vi "determinateTheRawSizeOfTable.vi"(0 "tableName":string, 3 "error in":errorcluster) -> (7 "sizeOfTableInNumberRaw":i32, 10 "error out":errorcluster)   [LabVIEW 2014]
uses:
  <vilib>/addons/database/Connection.llb/DB Tools Open Connec (String).vi
  <vilib>/addons/database/Connection.llb/Conn Execute.vi
  <vilib>/addons/database/Recordset.llb/Rec Fetch Integer Data (R).vi
  <vilib>/addons/database/Recordset.llb/Rec Destroy - Connection.vi
  <vilib>/addons/database/NI_Database_API.lvlib
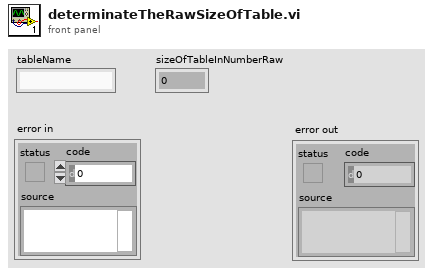
[diagram p1: front panel]
types:
  T1 = typedef "NI_Database_API.lvlib/Conn ObjectReference.ctl" = refnum<k1>
  T2 = typedef "NI_Database_API.lvlib/Rec ObjectReference.ctl" = refnum<k1>
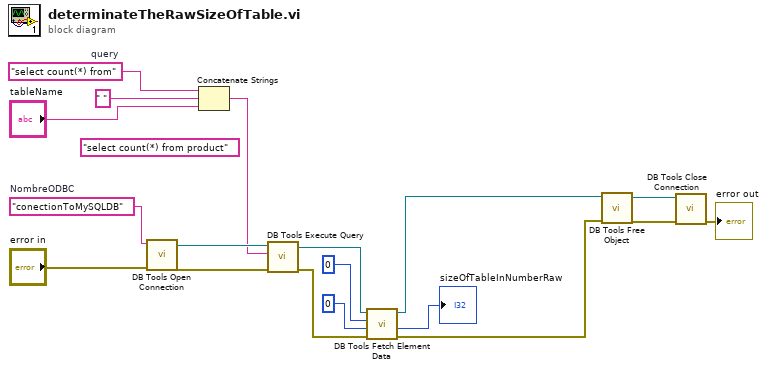
[diagram p0: block diagram]
diagram:
  w3 = "select count(*) from"  # query
  (unwired) "select count(*) from product" ("condition")
  w18 = "conectionToMySQLDB"  # NombreODBC
  n1 = call-poly <vilib>:"DB Tools Open Connection.vi"("error in (no error)"="error in", "connection information"=w18) -> ("error out"=w15:errorcluster, "connection reference"=w16:T1)  [unwired: 6 in]
  n2 = Concatenate Strings(w3, " " ("string"), "tableName") -> (w2:string)
  n3 = call-poly <vilib>:"DB Tools Execute Query.vi"("error in (no error)"=w15, "SQL query"=w2, "connection reference"=w16) -> ("error out"=w9:errorcluster, "recordset reference"=w12:T2)  [unwired: 5 in]
  n4 = call-poly <vilib>:"DB Tools Fetch Element Data.vi"("error in (no error)"=w9, "type"=0, "column index"=0, "recordset reference"=w12) -> ("error out"=w8:errorcluster, "data"=→"sizeOfTableInNumberRaw":i32, "recordset reference out"=w6:T2)  [unwired: 3 in]
  n5 = call-poly <vilib>:"DB Tools Free Object.vi"("error in (no error)"=w8, "recordset reference"=w6) -> ("error out"=w13:errorcluster, "connection reference"=w14:T1)  [unwired: 8 in]
  n6 = call <vilib>:"DB Tools Close Connection.vi"("error in (no error)"=w13, "connection reference"=w14) -> ("error out"=→"error out":errorcluster)  [unwired: 5 in]
